vi "pmu_Buffer Zero-crossing Frequencies.vi"(7 "Reset? (F)":bool, 9 "nominal Fs/actual Fs":dbl, 10 "timestamps out":dbl[](array[numeric]), 11 "frequencies":dbl[](array[numeric])) -> (3 "buffered zero-crossing frequency":T1)   [LabVIEW 2013, in "NI_EP_PMU.lvlib"]
uses:
  <vilib>/addons/Electrical Power/PMU/NI_EP_PMU.lvlib
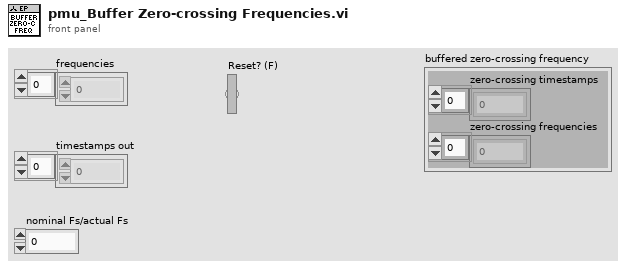
[diagram p1: front panel]
types:
  T1 = cluster{"zero-crossing timestamps":dbl[], "zero-crossing frequencies":dbl[]}
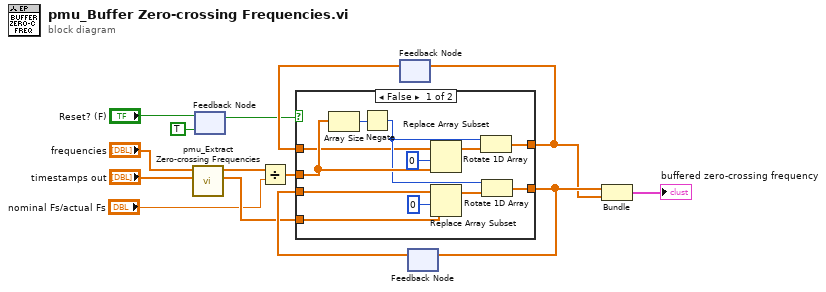
[diagram p0: block diagram]
diagram:
  n1 = call <vilib>:"pmu_Extract Zero-crossing Frequencies.vi"("timestamps in"="timestamps out", "frequencies in"="frequencies") -> ("zero-crossing timestamps"=w9:dbl[], "zero-crossing frequencies"=w3:dbl[])  [unwired: 8 in]
  n2 = feedback #1(TRUE) -> (w5:bool)
  n3 = feedback-in #1("Reset? (F)") -> ()
  n4 = Divide(x=w3, y="nominal Fs/actual Fs") -> (x/y=w4:dbl[])
  n5 = feedback #2() -> (w11:dbl[])  [unwired: 1 in]
  n6 = feedback #3() -> (w13:dbl[])  [unwired: 1 in]
  n7 = case shown="False" w5 {
    tunnel: w9 -> [w22 w27]
    tunnel: w4 -> [w21 w28]
    tunnel: [w18 w27] -> w12
    tunnel: [w17 w28] -> w1
    tunnel: w11 -> [w16 _]
    tunnel: w13 -> [w15 _]
    frame False {
      n8 = Array Size(array=w21) -> (size(s)=w20:i32)
      n9 = Negate(x=w20) -> (-x=w19:i32)
      n10 = Replace Array Subset(array=w16, new element=w21, index=0) -> (w26:dbl[])
      n11 = Replace Array Subset(array=w15, new element=w22, index=0) -> (w23:dbl[])
      n12 = Rotate 1D Array(1:w26, 2:w19) -> (0:w17:dbl[])
      n13 = Rotate 1D Array(1:w23, 2:w19) -> (0:w18:dbl[])
    }
    frame True {
    }
  }
  n14 = feedback-in #2(w1) -> ()
  n15 = feedback-in #3(w12) -> ()
  n16 = Bundle("zero-crossing timestamps"=w12, w1) -> (→"buffered zero-crossing frequency":cluster{"zero-crossing timestamps":dbl[], dbl[]})  [unwired: 1 in]
